vi "sg Set Custom IQ.vi"(0 "device":i32, 1 "length":i32, 5 "clockRate":dbl, 7 "IVals":dbl, 9 "QVals":dbl, 11 "error in (no error)":errorcluster, 12 "period":i32) -> (4 "function return":u32(ring), 8 "IVals out":dbl, 10 "QVals out":dbl, 15 "error out":errorcluster)   [LabVIEW 2014, in "VSG25A.lvlib"]
doc: "SG_API sgStatus sgSetCustomIQ(int device, double clockRate, double *IVals,\n double *QVals, int length, int period);"
uses:
  VSG25A.lvlib
  sg_api.dll
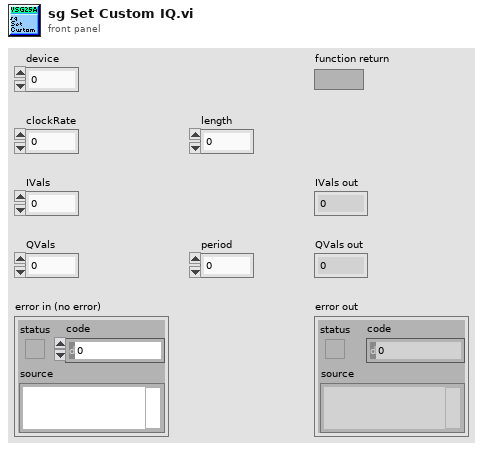
[diagram p1: front panel]
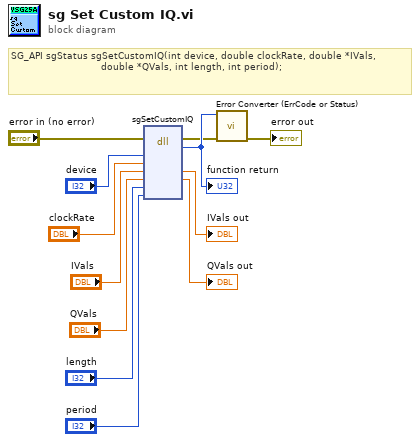
[diagram p0: block diagram]
diagram:
  # "SG_API sgStatus sgSetCustomIQ(int device, double clockRate, double *IVals,\n                              double *QVals, int length, int period);"
  n1 = dll-call lib="C:/Users/M_LAPTOP/Desktop/Labview/practice/VSG25A/sg_lib/sg_api.*" fn="sgSetCustomIQ"(error in="error in (no error)", "device"="device", "clockRate"="clockRate", "IVals"="IVals", "QVals"="QVals", "length"="length", "period"="period") -> (error out=w2:errorcluster, w12:u32, "IVals"=→"IVals out":dbl, "QVals"=→"QVals out":dbl)  [unwired: 6 in, 1 out]
  "function return" <- w12
  n2 = call "Error Converter (ErrCode or Status).vi"("error in (no error)"=w2, "error code"=w12) -> ("error out"=→"error out":errorcluster)  [unwired: 9 in]
